vi "Clock Deriver.vi"(9 "Reset":bool, 11 "Divisor":u32=1 min=1) -> (2 "Clock Out":bool)   [LabVIEW 2010]
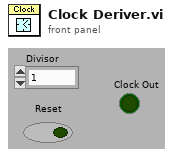
[diagram p1: front panel]
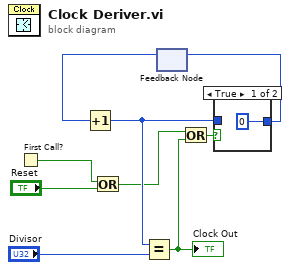
[diagram p0: block diagram]
diagram:
  n1 = First Call?() -> (First Call?: T/F=w1:bool)
  n2 = Or(x=w1, y="Reset") -> (x .or. y?=w2:bool)
  n3 = feedback #1() -> (w5:u32)  [unwired: 1 out]
  n4 = Increment(x=w5) -> (x+1=w4:u32)
  n5 = Equal?(x=w4, y="Divisor") -> (x = y?=w6:bool)
  "Clock Out" <- w6
  n6 = Or(x=w2, y=w6) -> (x .or. y?=w9:bool)
  n7 = case shown="True" w9 {
    tunnel: [u32 0 w11] -> w3
    tunnel: w4 -> [_ w11]
    frame True {
    }
    frame False {
    }
  }
  n8 = feedback-in #1(w3) -> ()
